vi "Example_CircularBuffer.vi"() -> ()   [LabVIEW 2024]
uses:
  TypedCircularBuffer.lvclass
  Type.ctl
panel:
  out "Copied Buffer":T1[](array[typedef])
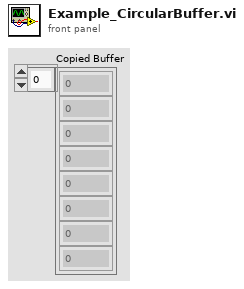
[diagram p1: front panel]
types:
  T1 = typedef "TypedCircularBuffer.lvclass/Type.ctl" = i32
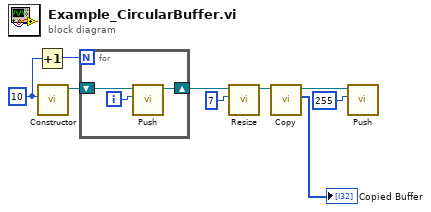
[diagram p0: block diagram]
diagram:
  w9 = u32 10 ("Capacity")
  n1 = Increment(x=w9) -> (x+1=w8:u32)
  n2 = call "Constructor.vi"("Capacity"=w9) -> ("TypedCircularBuffer out"=w7:refnum<class "TypedCircularBuffer.lvclass">)  [unwired: 10 in]
  n3 = for {
    N: w8 -> [_]
    shift-right: [w11] -> w5
    shift-left: w7 -> [w12]
    i -> [w10]
    n4 = call "Push.vi"("Element"=w10, "TypedCircularBuffer in"=w12) -> ("TypedCircularBuffer out"=w11:refnum<class "TypedCircularBuffer.lvclass">)  [unwired: 7 in, 2 out]
  }
  n5 = call "Resize.vi"("Capacity"=u32 7, "TypedCircularBuffer in"=w5) -> ("TypedCircularBuffer out"=w4:refnum<class "TypedCircularBuffer.lvclass">)  [unwired: 9 in]
  n6 = call "Copy.vi"("TypedCircularBuffer in"=w4) -> ("Copied Buffer"=→"Copied Buffer":T1[], "TypedCircularBuffer out"=w2:refnum<class "TypedCircularBuffer.lvclass">)  [unwired: 9 in]
  n7 = call "Push.vi"("Element"=u8 255, "TypedCircularBuffer in"=w2) -> ()  [unwired: 7 in, 3 out]
